vi "FTW-TestSupport-Actor-EchoServer.vi"(0 "Actor Instance Configuration":string="{\n  \"Identity\": \"ActorName\",\n  \"InboxAddress\": \"tcp://127.0.0.1:*\",\n  \"SupervisorAddress\": \"\",\n  \"DebugEnableInboxLogging\": false,\n  \"DebugEnableJobLogging\": false,\n  \"DebugShowPanel\": false\n}", 5 "Idle Timeout":i32=1000 format="%d msec", 11 "ErrorIn":errorcluster) -> (15 "Error":errorcluster)   [LabVIEW 2015]
uses:
  src/actor/instance/FTW-Actor-Instance.lvclass
panel:
  # "Inputs"
  # "Outputs"
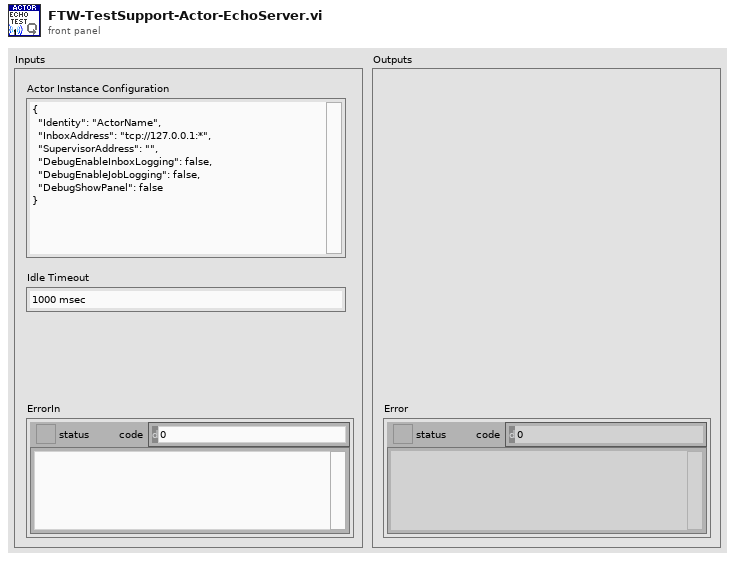
[diagram p1: front panel]
types:
  T1 = cluster{"Incoming Request":refnum<event-registration>}
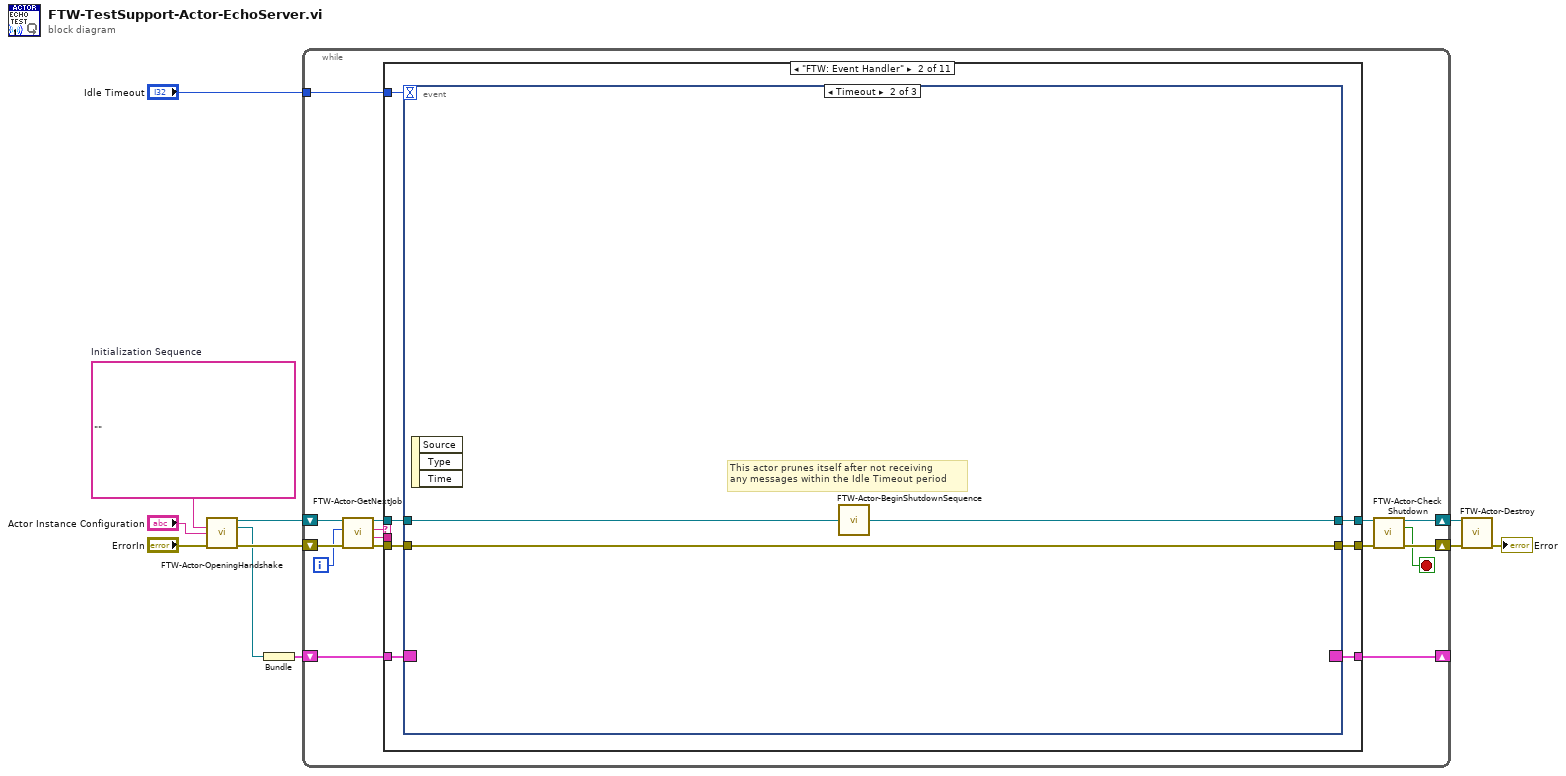
[diagram p0: block diagram]
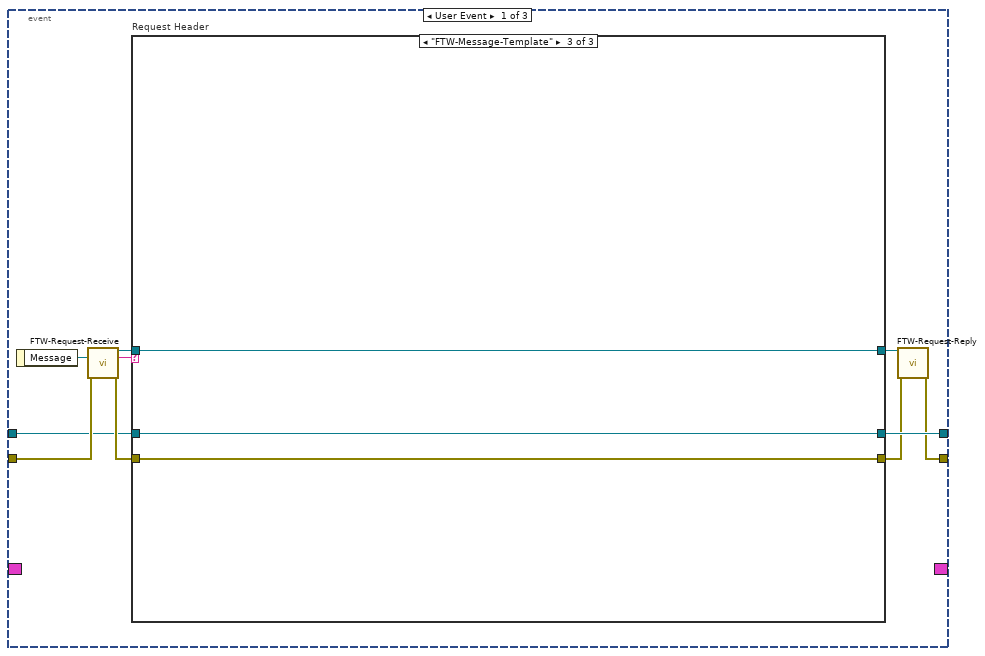
[diagram p3: hidden frame]
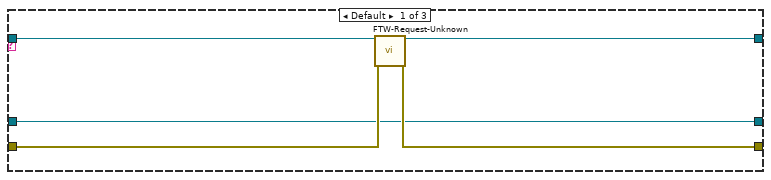
[diagram p4: hidden frame]
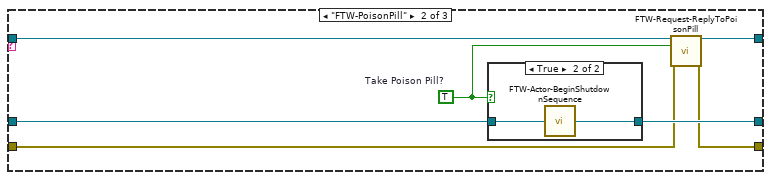
[diagram p5: hidden frame]
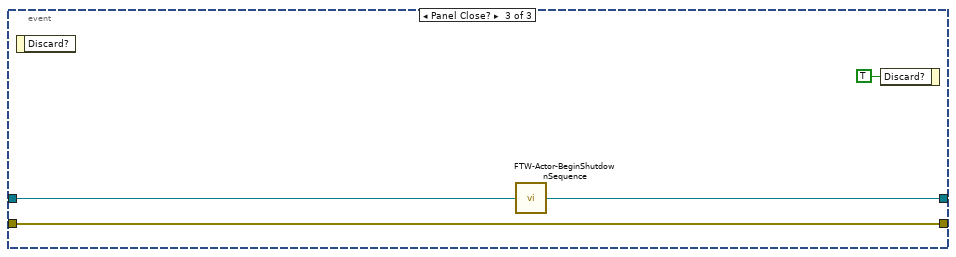
[diagram p7: hidden frame]
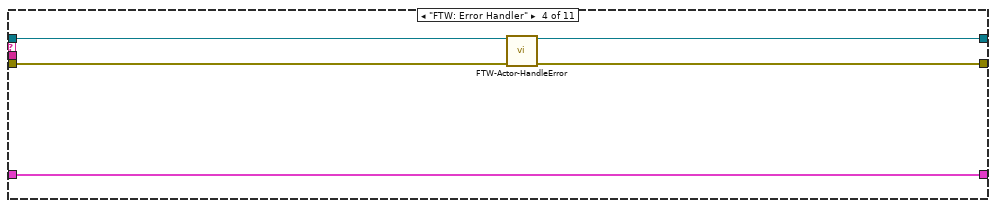
[diagram p9: hidden frame]
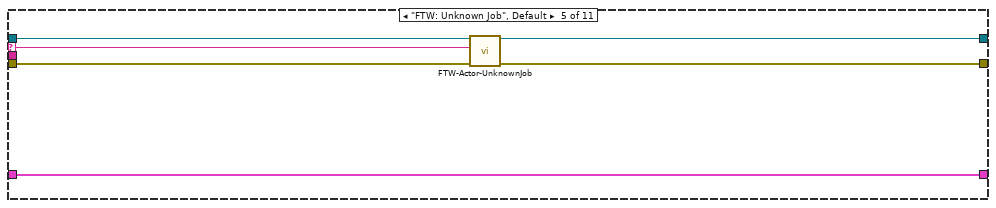
[diagram p10: hidden frame]
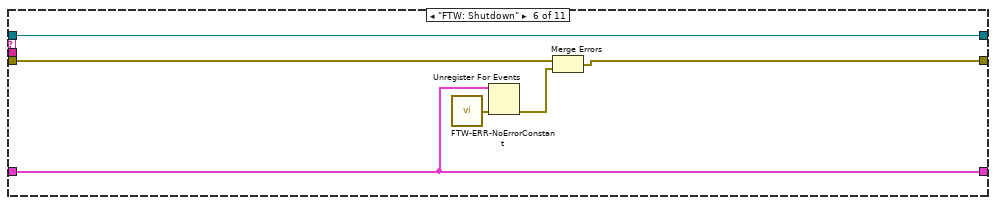
[diagram p11: hidden frame]
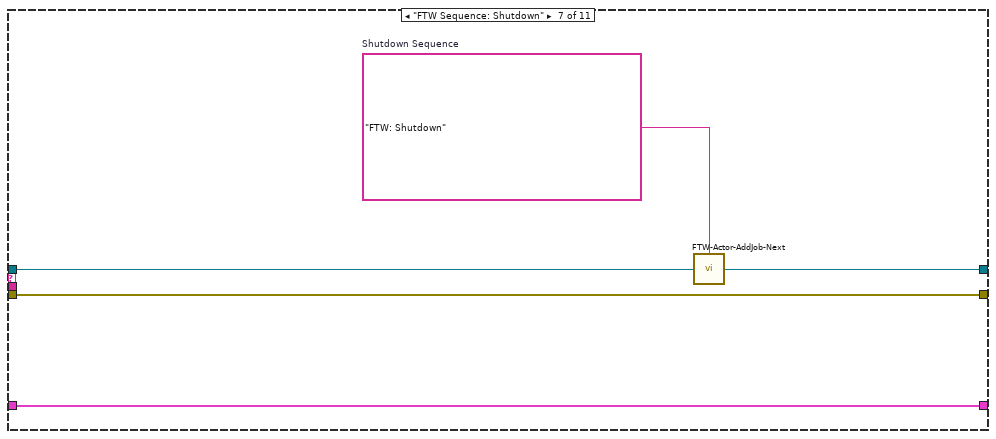
[diagram p12: hidden frame]
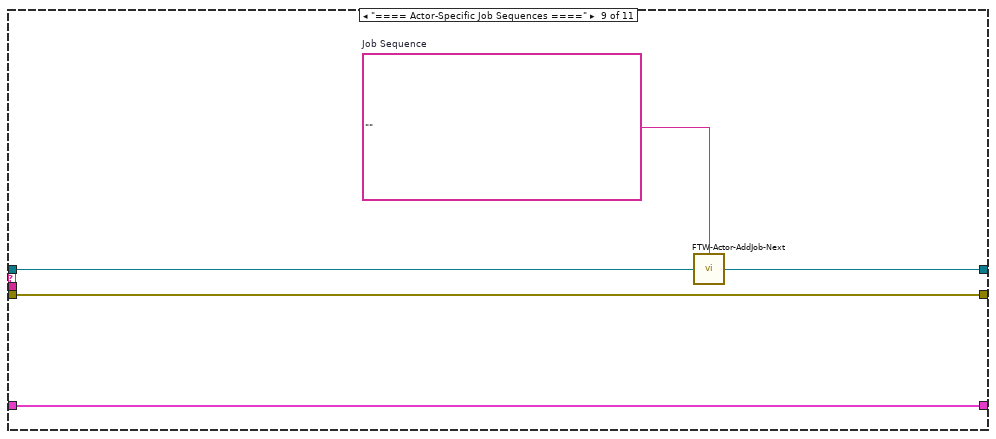
[diagram p14: hidden frame]
diagram:
  w6 = ""  # Initialization Sequence
  n1 = call "FTW-Actor-OpeningHandshake.vi"("Initialization Job Sequence"=w6, "Actor Instance Configuration"="Actor Instance Configuration", "error in"="ErrorIn") -> ("FTW Actor Instance"=w11:refnum<class "FTW-Actor-Instance.lvclass">, "Incoming Request"=w2:refnum<event-registration>, "error out"=w7:errorcluster)  [unwired: 10 in]
  n2 = Bundle("Incoming Request"=w2) -> (w4:T1)  [unwired: 1 in]
  n3 = while {
    shift-right: [w16] -> w9
    shift-left: w7 -> [w23]
    shift-right: [w13] -> _
    shift-left: w4 -> [w26]
    shift-right: [w18] -> w10
    shift-left: w11 -> [w25]
    tunnel: "Idle Timeout" -> [w12]
    i -> [w14]
    stop <- w15 stop-if-true
    n4 = call "FTW-Actor-GetNextJob.vi"("error in"=w23, "Jobs Performed"=w14, "FTW Actor Instance"=w25) -> ("error out"=w22:errorcluster, "Job Data"=w20:string, "Job Name"=w21:string, "FTW Actor Instance out"=w24:refnum<class "FTW-Actor-Instance.lvclass">)  [unwired: 5 in]
    n5 = case shown="\"FTW: Event Handler\"" w21 {
      selector: w21 -> [_ _ _ _ w80 _ _ _ _ _ _]
      tunnel: [w28 w36 w72 w75 w83 w90 w95 w98 w103 w107 w110] -> w17
      tunnel: w22 -> [w28 w35 w72 w77 w84 w91 w95 w98 w103 w107 w110]
      tunnel: w26 -> [w29 w31 w74 w79 w85 w87 w96 w99 w104 w106 w109]
      tunnel: [w29 w34 w74 w79 w85 w87 w96 w99 w104 w106 w109] -> w13
      tunnel: w20 -> [_ _ _ _ _ _ _ _ _ _ _]
      tunnel: [w27 w33 w73 w76 w81 w88 w93 w97 w101 w105 w108] -> w19
      tunnel: w24 -> [w27 w32 w73 w78 w82 w88 w94 w97 w102 w105 w108]
      tunnel: w12 -> [_ w30 _ _ _ _ _ _ _ _ _]
      frame "==== Featherweight Framework Jobs ====" {
      }
      frame "FTW: Event Handler" {
        n6 = event shown="[1] Timeout" {
          selector: w31 -> [_ _ _]
          dyn-events: [_ _ _] -> w34
          timeout: w30 -> [_ _ _]
          tunnel: [w40 w67 w70] -> w36
          tunnel: w35 -> [w45 w67 w70]
          tunnel: [w44 w65 w68] -> w33
          tunnel: w32 -> [w43 w66 w69]
          event User Event {
            n7 = event-data() -> ("Message"=w37:refnum<queue>)  [unwired: 1 in]
            n8 = call "FTW-Request-Receive.vi"("MessagePipe"=w37, "error in"=w45) -> ("Request"=w41:refnum<data-value>, "Request Header"=w42:string, "error out"=w46:errorcluster)  [unwired: 11 in]
            n9 = case "Request Header" shown="\"FTW-Message-Template\"" w42 {
              tunnel: [w50 w53 w62] -> w39
              tunnel: w46 -> [w51 w54 w62]
              tunnel: [w48 w58 w64] -> w44
              tunnel: w43 -> [w48 w57 w64]
              tunnel: w41 -> [w49 w56 w63]
              tunnel: [w47 w55 w63] -> w38
              frame Default {
                n10 = call "FTW-Request-Unknown.vi"("Request"=w49, "error in"=w51) -> ("Request out"=w47:refnum<data-value>, "error out"=w50:errorcluster)  [unwired: 12 in]
              }
              frame "FTW-PoisonPill" {
                w52 = TRUE  # Take Poison Pill?
                n11 = case shown="True" w52 {
                  tunnel: [w59 w61] -> w58
                  tunnel: w57 -> [w59 w60]
                  frame False {
                  }
                  frame True {
                    n12 = call "FTW-Actor-BeginShutdownSequence.vi"("FTW Actor Instance"=w60) -> ("FTW Actor Instance out"=w61:refnum<class "FTW-Actor-Instance.lvclass">)  [unwired: 3 in]
                  }
                }
                n13 = call "FTW-Request-ReplyToPoisonPill.vi"("Poison Pill Request"=w56, "Shutting Down?"=w52, "error in"=w54) -> ("Poison Pill Response"=w55:refnum<data-value>, "error out"=w53:errorcluster)  [unwired: 11 in]
              }
              frame "FTW-Message-Template" {
              }
            }
            n14 = call "FTW-Request-Reply.vi"("Request"=w38, "error in"=w39) -> ("error out"=w40:errorcluster)  [unwired: 13 in]
          }
          event Timeout {
            # "This actor prunes itself after not receiving\nany messages within the Idle Timeout period"
            n15 = event-data() -> ()  [unwired: 1 in, 3 out]
            n16 = call "FTW-Actor-BeginShutdownSequence.vi"("FTW Actor Instance"=w66) -> ("FTW Actor Instance out"=w65:refnum<class "FTW-Actor-Instance.lvclass">)  [unwired: 3 in]
          }
          event Panel Close? {
            n17 = event-data() -> ()  [unwired: 1 in, 1 out]
            n18 = call "FTW-Actor-BeginShutdownSequence.vi"("FTW Actor Instance"=w69) -> ("FTW Actor Instance out"=w68:refnum<class "FTW-Actor-Instance.lvclass">)  [unwired: 3 in]
            n19 = event-data("Discard?"=TRUE) -> ()  [unwired: 1 in, 1 out]
          }
        }
      }
      frame "FTW: Failure to Launch" {
      }
      frame "FTW: Error Handler" {
        n20 = call-dynamic "FTW-Actor-HandleError.vi"("FTW Actor Instance"=w78, "error in"=w77) -> ("FTW Actor Instance out"=w76:refnum<class "FTW-Actor-Instance.lvclass">, "error out"=w75:errorcluster)  [unwired: 11 in, 1 out]
      }
      frame "FTW: Unknown Job", Default {
        n21 = call-dynamic "FTW-Actor-UnknownJob.vi"("FTW Actor Instance"=w82, "Unknown Job"=w80, "error in"=w84) -> ("FTW Actor Instance out"=w81:refnum<class "FTW-Actor-Instance.lvclass">, "error out"=w83:errorcluster)  [unwired: 11 in]
      }
      frame "FTW: Shutdown" {
        n22 = call "FTW-ERR-NoErrorConstant.vi"() -> ("no error"=w86:errorcluster)
        n23 = Unregister For Events(event registration refnum=w87, error in=w86) -> (error out=w89:errorcluster)
        n24 = Merge Errors(w91, w89) -> (w90:errorcluster)
      }
      frame "FTW Sequence: Shutdown" {
        w92 = "FTW: Shutdown"  # Shutdown Sequence
        n25 = call "FTW-Actor-AddJob-Next.vi"("Add Next in Job Queue"=w92, "FTW Actor Instance"=w94) -> ("FTW Actor Instance out"=w93:refnum<class "FTW-Actor-Instance.lvclass">)  [unwired: 2 in]
      }
      frame "==== Actor-Specific Static Dependencies ====" {
      }
      frame "==== Actor-Specific Job Sequences ====" {
        w100 = ""  # Job Sequence
        n26 = call "FTW-Actor-AddJob-Next.vi"("Add Next in Job Queue"=w100, "FTW Actor Instance"=w102) -> ("FTW Actor Instance out"=w101:refnum<class "FTW-Actor-Instance.lvclass">)  [unwired: 2 in]
      }
      frame "==== Actor-Specific Jobs ====" {
      }
      frame "ActorName: Job Template" {
      }
    }
    n27 = call "FTW-Actor-CheckShutdown.vi"("FTW Actor Instance"=w19, "error in"=w17) -> ("FTW Actor Instance out"=w18:refnum<class "FTW-Actor-Instance.lvclass">, "Shutdown?"=w15:bool, "error out"=w16:errorcluster)  [unwired: 11 in]
  }
  n28 = call-dynamic "FTW-Actor-Destroy.vi"("FTW Actor Instance"=w10, "error in"=w9) -> ("error out"=→"Error":errorcluster)  [unwired: 13 in]
